vi "KolejkaMycia.vi"(8 "error in (no error)":errorcluster, 11 "Wash Options":T1) -> (0 "error out":errorcluster, 3 "Option Array":string[](array[string]))   [LabVIEW 2020]
uses:
  controls/WashOptions.ctl
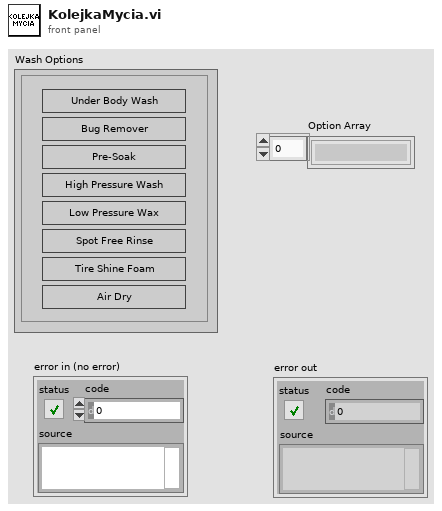
[diagram p1: front panel]
types:
  T1 = typedef "WashOptions.ctl" = cluster{"Bug Remover":bool, "Low Pressure Wax":bool, "High Pressure Wash":bool, "Pre-Soak":bool, "Spot Free Rinse":bool, "Air Dry":bool, "Under Body Wash":bool, "Tire Shine Foam":bool}
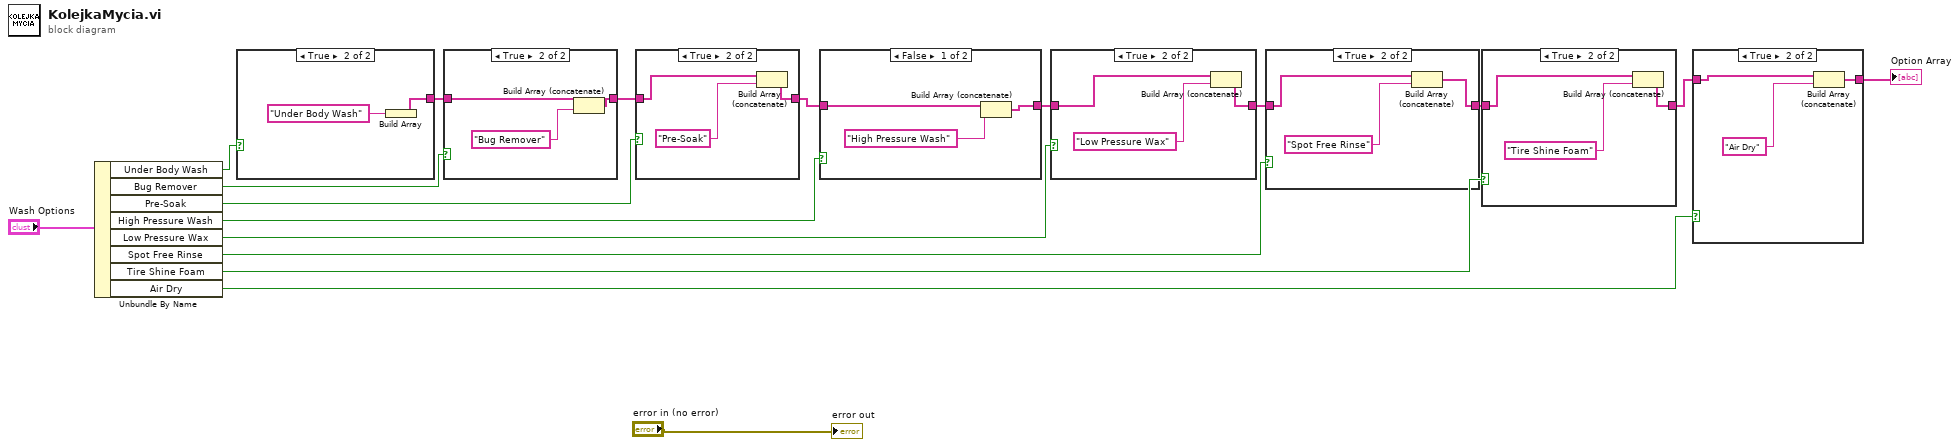
[diagram p0: block diagram]
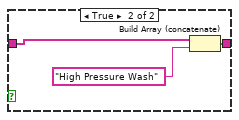
[diagram p6: hidden frame]
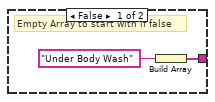
[diagram p9: hidden frame]
diagram:
  n1 = Unbundle By Name("Wash Options") -> ("Under Body Wash"=w11:bool, "Bug Remover"=w17:bool, "Pre-Soak"=w18:bool, "High Pressure Wash"=w16:bool, "Low Pressure Wax"=w15:bool, "Spot Free Rinse"=w14:bool, "Tire Shine Foam"=w13:bool, "Air Dry"=w12:bool)
  n2 = case shown="True" w11 {
    tunnel: [w19 w21] -> w6
    frame False {
      # "Empty Array to start with if false"
      n3 = Build Array("Under Body Wash") -> (w19:string[])
    }
    frame True {
      n4 = Build Array("Under Body Wash") -> (w21:string[])
    }
  }
  n5 = case shown="True" w17 {
    tunnel: w6 -> [w23 w25]
    tunnel: [w23 w24] -> w5
    frame False {
    }
    frame True {
      n6 = Build Array (concatenate)(w25, "Bug Remover") -> (w24:string[])
    }
  }
  n7 = case shown="True" w18 {
    tunnel: w5 -> [w27 w29]
    tunnel: [w27 w28] -> w4
    frame False {
    }
    frame True {
      n8 = Build Array (concatenate)(w29, "Pre-Soak") -> (w28:string[])
    }
  }
  n9 = case shown="False" w16 {
    tunnel: [w31 w35] -> w10
    tunnel: w4 -> [w32 w34]
    frame False {
      n10 = Build Array (concatenate)(w32, "High Pressure Wash") -> (w31:string[])
    }
    frame True {
      n11 = Build Array (concatenate)(w34, "High Pressure Wash") -> (w35:string[])
    }
  }
  n12 = case shown="True" w15 {
    tunnel: w10 -> [w37 w40]
    tunnel: [w37 w38] -> w3
    frame False {
    }
    frame True {
      n13 = Build Array (concatenate)(w40, "Low Pressure Wax") -> (w38:string[])
    }
  }
  n14 = case shown="True" w14 {
    tunnel: w3 -> [w41 w43]
    tunnel: [w41 w42] -> w2
    frame False {
    }
    frame True {
      n15 = Build Array (concatenate)(w43, "Spot Free Rinse") -> (w42:string[])
    }
  }
  n16 = case shown="True" w13 {
    tunnel: w2 -> [w45 w47]
    tunnel: [w45 w46] -> w1
    frame False {
    }
    frame True {
      n17 = Build Array (concatenate)(w47, "Tire Shine Foam") -> (w46:string[])
    }
  }
  n18 = case shown="True" w12 {
    tunnel: [w49 w51] -> w8
    tunnel: w1 -> [w49 w50]
    frame False {
    }
    frame True {
      n19 = Build Array (concatenate)(w50, "Air Dry") -> (w51:string[])
    }
  }
  "Option Array" <- w8
  "error out" <- "error in (no error)"
